vi "Read Bootloader ID.vi"(6 "error in":errorcluster, 8 "MaxRead":i32, 9 "Channel in":u16) -> (0 "error out":errorcluster, 1 "Messages":T1(array[cluster]), 2 "Pass":bool, 3 "Channel out":u16, 4 "Bootloader ID":string)   [LabVIEW 2023]
uses:
  4f930f32-d09a-43ef-bca1-8b214b378bd5.vi
  e8470de1-fa2d-4ee3-b50e-96bd89dc731f.vi
  d0f02419-cfb7-4a5e-bc3c-f035efdb0e96.vi
  Communication/PCAN2023/PCAN API.lvlib
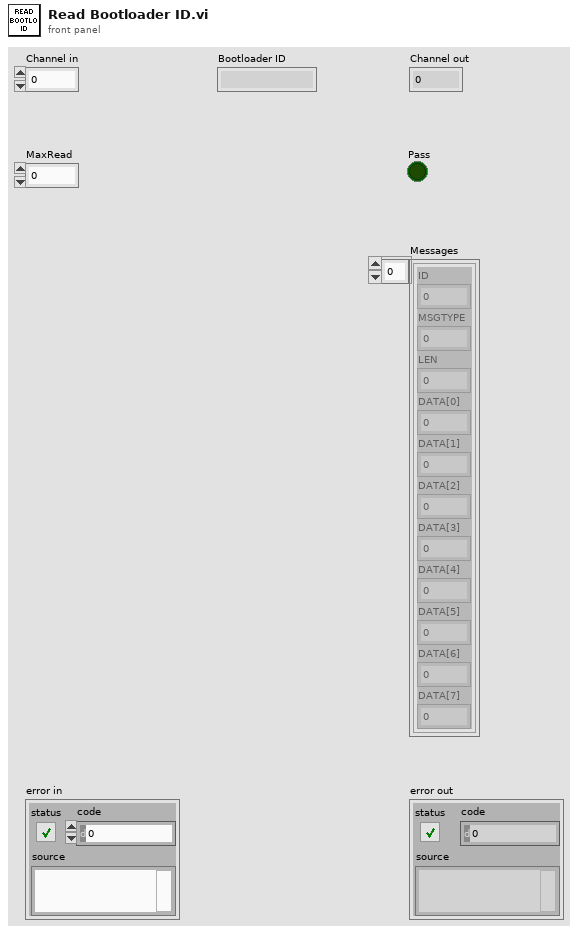
[diagram p1: front panel]
types:
  T1 = cluster{"ID":u32, "MSGTYPE":u8, "LEN":u8, "DATA[0]":u8, "DATA[1]":u8, "DATA[2]":u8, "DATA[3]":u8, "DATA[4]":u8, "DATA[5]":u8, "DATA[6]":u8, "DATA[7]":u8}[]
  T2 = cluster{"ID":u32, "MSGTYPE":u8, "LEN":u8, "DATA[0]":u8, "DATA[1]":u8, "DATA[2]":u8, "DATA[3]":u8, "DATA[4]":u8, "DATA[5]":u8, "DATA[6]":u8, "DATA[7]":u8}
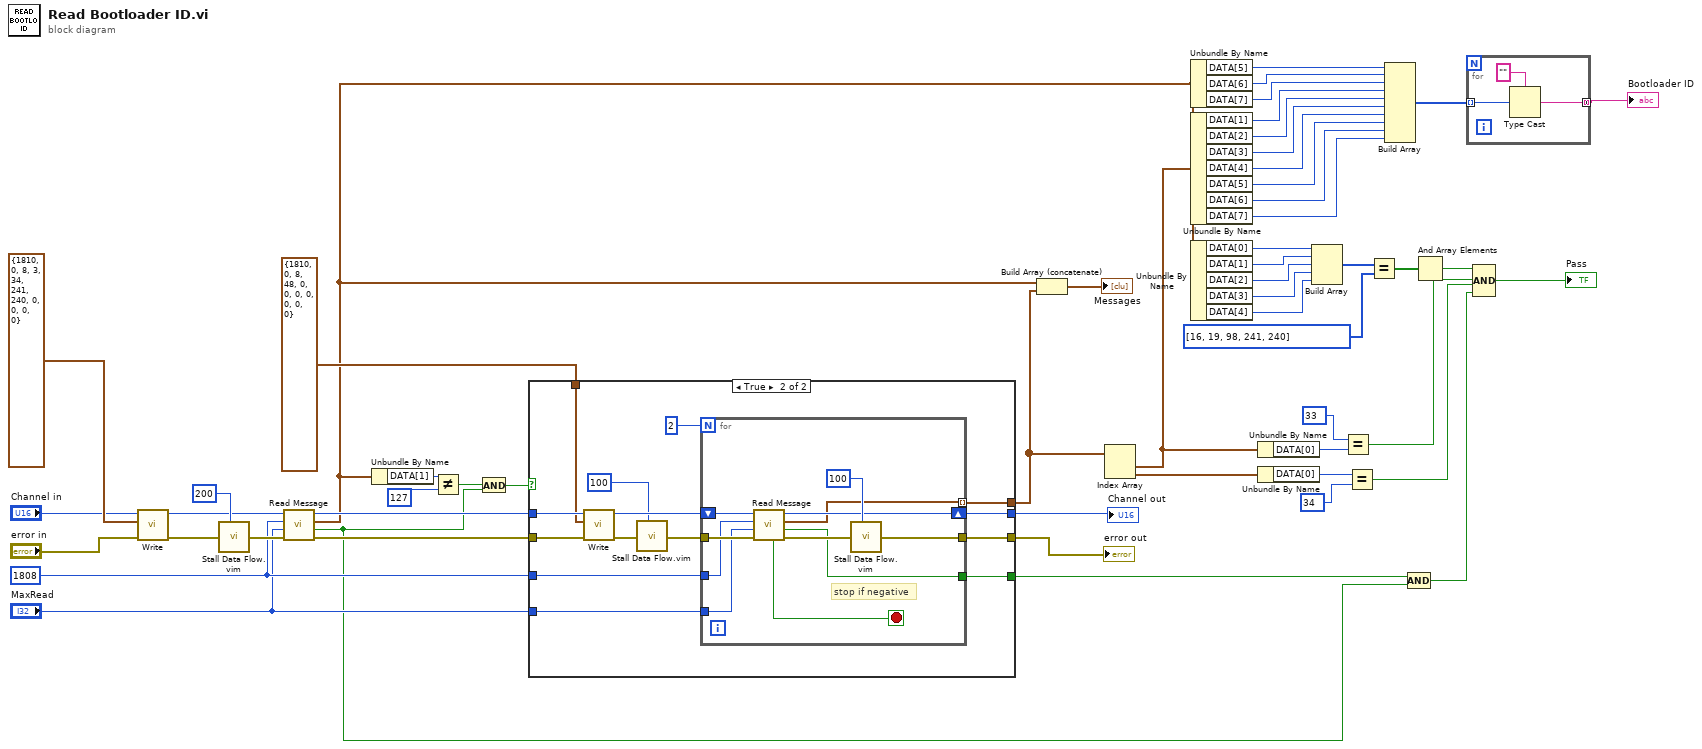
[diagram p0: block diagram]
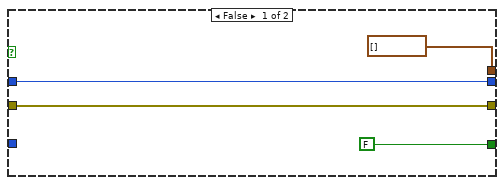
[diagram p2: hidden frame]
diagram:
  (unwired) u32 200 ("milliseconds to wait")
  w5 = u32 1808 ("ID")
  n1 = call "Write.vi"("error in"="error in", "MessageBuffer"=T2 {"ID"=1810, "MSGTYPE"=0, "LEN"=8, "DATA[0]"=3, "DATA[1]"=34, "DATA[2]"=241, "DATA[3]"=240, "DATA[4]"=0, "DATA[5]"=0, "DATA[6]"=0, "DATA[7]"=0}, "Channel"="Channel in") -> ("error out"=w50:errorcluster, "Channel out"=w10:u16)  [unwired: 5 in, 2 out]
  n2 = call "Stall Data Flow.vim"("value in"=w50, "milliseconds to wait"=u32 200) -> ("value out"=w8:errorcluster)  [unwired: 1 out]
  n3 = call "Read Message.vi"("error in"=w8, "MaxRead"="MaxRead", "ID"=w5, "Channel in"=w10) -> ("error out"=w7:errorcluster, "Passed"=w1:bool, "Last Message"=w6:T2, "Channel out"=w9:u16)  [unwired: 3 in, 1 out]
  n4 = Unbundle By Name(w6) -> ("DATA[1]"=w45:u8)
  n5 = Not Equal?(x=w45, y=u8 127) -> (x != y?=w3:bool)
  n6 = And(x=w3, y=w1) -> (x .and. y?=w2:bool)
  n7 = case shown="True" w2 {
    tunnel: w9 -> [w57 w72]
    tunnel: w7 -> [w55 w71]
    tunnel: [w55 w70] -> w49
    tunnel: [FALSE w69] -> w48
    tunnel: [w57 w67] -> w47
    tunnel: T2 {"ID"=1810, "MSGTYPE"=0, "LEN"=8, "DATA[0]"=48, "DATA[1]"=0, "DATA[2]"=0, "DATA[3]"=0, "DATA[4]"=0, "DATA[5]"=0, "DATA[6]"=0, "DATA[7]"=0} ("MessageBuffer") -> [_ w65]
    tunnel: [T1 [] w61] -> w17
    tunnel: w5 -> [_ w60]
    tunnel: "MaxRead" -> [_ w59]
    frame False {
    }
    frame True {
      n8 = call "Write.vi"("error in"=w71, "MessageBuffer"=w65, "Channel"=w72) -> ("error out"=w62:errorcluster, "Channel out"=w68:u16)  [unwired: 5 in, 2 out]
      n9 = call "Stall Data Flow.vim"("value in"=w62, "milliseconds to wait"=u32 100) -> ("value out"=w66:errorcluster)  [unwired: 1 out]
      n10 = for {
        N: 2 -> [_]
        tunnel: [w76] -> w69
        shift-right: [w80] -> w67
        shift-left: w68 -> [w81]
        tunnel: w66 -> [w79]
        tunnel: [w83] -> w70
        tunnel: [w77] -> w61 mode=indexing
        tunnel: w60 -> [w74]
        tunnel: w59 -> [w73]
        stop <- w75 stop-if-true
        # "stop if negative"
        n11 = call "Read Message.vi"("error in"=w79, "MaxRead"=w73, "ID"=w74, "Channel in"=w81) -> ("error out"=w78:errorcluster, "Passed"=w76:bool, "Last Message"=w77:T2, "Channel out"=w80:u16, "Negative"=w75:bool)  [unwired: 3 in]
        n12 = call "Stall Data Flow.vim"("value in"=w78, "milliseconds to wait"=u32 100) -> ("value out"=w83:errorcluster)  [unwired: 1 out]
      }
    }
  }
  "error out" <- w49
  "Channel out" <- w47
  n13 = Build Array (concatenate)(w6, w17) -> (→"Messages":T1)
  n14 = Index Array(array=w17) -> (element #1=w15:T2, element #2=w16:T2)  [unwired: 2 in]
  n15 = Unbundle By Name(w6) -> ("DATA[5]"=w27:u8, "DATA[6]"=w26:u8, "DATA[7]"=w25:u8)
  n16 = Unbundle By Name(w15) -> ("DATA[1]"=w22:u8, "DATA[2]"=w21:u8, "DATA[3]"=w20:u8, "DATA[4]"=w19:u8, "DATA[5]"=w18:u8, "DATA[6]"=w12:u8, "DATA[7]"=w11:u8)
  n17 = Unbundle By Name(w6) -> ("DATA[0]"=w42:u8, "DATA[1]"=w41:u8, "DATA[2]"=w40:u8, "DATA[3]"=w39:u8, "DATA[4]"=w38:u8)
  n18 = Unbundle By Name(w15) -> ("DATA[0]"=w35:u8)
  n19 = Unbundle By Name(w16) -> ("DATA[0]"=w32:u8)
  n20 = Build Array(w42, w41, w40, w39, w38) -> (w37:u8[])
  n21 = Equal?(x=u8 33, y=w35) -> (x = y?=w30:bool)
  n22 = Equal?(x=w32, y=u8 34 ("x")) -> (x = y?=w28:bool)
  n23 = Equal?(x=w37, y=u8[] [16, 19, 98, 241, 240]) -> (x = y?=w31:bool[])
  n24 = Build Array(w27, w26, w25, w22, w21, w20, w19, w18, w12, w11) -> (w24:u8[])
  n25 = Compound Arithmetic op=AND(w48, w1) -> (w13:bool)
  n26 = And Array Elements(Boolean array=w31) -> (logical AND=w29:bool)
  n27 = for {
    tunnel: w24 -> [w85] mode=indexing
    tunnel: [w84] -> w23 mode=concatenating
    n28 = Type Cast(type="", x=w85) -> (*(type *) &x=w84:string)
  }
  "Bootloader ID" <- w23
  n29 = Compound Arithmetic op=AND(w29, w30, w28, w13) -> (→"Pass":bool)
